vi "CtrlTrain_Analog_HighSelect.vi"(8 "Input_4":dbl=-9.9e+30, 9 "Input_3":dbl=-9.9e+30, 10 "Input_2":dbl=-9.9e+30, 11 "Input_1":dbl=-9.9e+30) -> (3 "Output":dbl)   [LabVIEW 2019, in "CtrlTrainingLibary_Protected.lvlib"]
doc: "This VI rate limits the input. This VI remembers the last output. If there are multiple VI that set the same output, use the RateLimit2 VI. This one has an input connection to send the last output value."
uses:
  CtrlTrainingLibary_Protected.lvlib
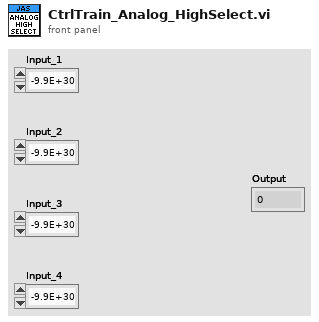
[diagram p1: front panel]
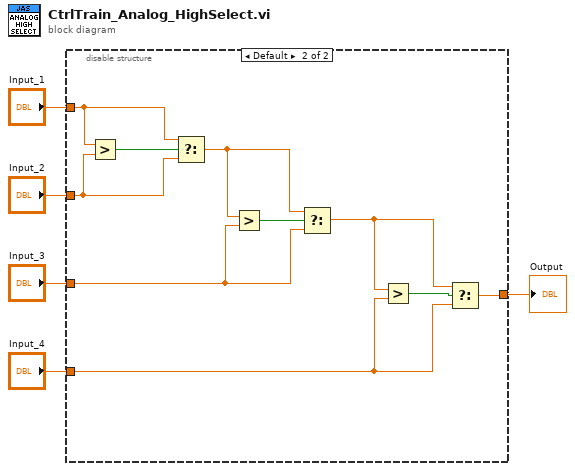
[diagram p0: block diagram]
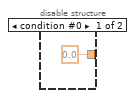
[diagram p2: hidden frame]
diagram:
  n1 = disable-structure shown="Default" {
    disable-tunnel: "Input_1" -> [_ w15]
    disable-tunnel: "Input_2" -> [_ w14]
    disable-tunnel: "Input_4" -> [_ w10]
    disable-tunnel: "Input_3" -> [_ w9]
    disable-tunnel: [0.0 ("Input_4") w8] -> w1
    frame condition #0 {
    }
    frame condition #1 (active) {
      n2 = Greater?(x=w15, y=w14) -> (0:w16:bool)
      n3 = Select(t=w15, s=w16, f=w14) -> (s? t:f=w12:dbl)
      n4 = Greater?(x=w12, y=w9) -> (0:w13:bool)
      n5 = Select(t=w12, s=w13, f=w9) -> (s? t:f=w7:dbl)
      n6 = Greater?(x=w7, y=w10) -> (0:w11:bool)
      n7 = Select(t=w7, s=w11, f=w10) -> (s? t:f=w8:dbl)
    }
  }
  "Output" <- w1
